vi "总氮流程质控自动启动.vi"(10 "总氮量程切换":enum32{"H", "L", "AUTO"}(ring)=enum."AUTO", 11 "参数":T1={"是否启用仪器"=FALSE, "CODMn"={"启动测量模式"={"测量模式"=enum."水样测量"}, "确定按钮"=TRUE}, "启动模块"={"氨氮"=FALSE, "总磷"=FALSE, "总氮"=FALSE, "COD"=FALSE}, "常规启动"=FALSE, "直接启动"=FALSE}) -> ()   [LabVIEW 2016]
panel:
  out "枚举 2":enum16{"初始化", "采配水启动", "等待", "配水", "排水", "结束"}(ring)
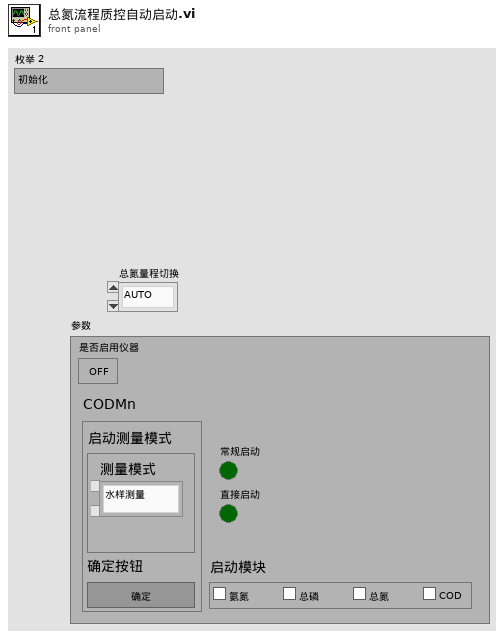
[diagram p1: front panel]
types:
  T1 = cluster{"是否启用仪器":bool, "CODMn":cluster{"启动测量模式":cluster{"测量模式":enum16{"水样测量", "标样核查", "加标回收", "平行样", "校零", "校标"}}, "确定按钮":bool}, "启动模块":cluster{"氨氮":bool, "总磷":bool, "总氮":bool, "COD":bool}, "常规启动":bool, "直接启动":bool}
  T2 = cluster{"R0":i16, "R1":i16, "R2":i16, "R3":i16, "R4":i16, "R5":i16, "R6":i16, "R7":i16, "R8":i16, "R9":i16, "R10":i16, "R11":i16, "R12":i16, "R13":i16, "R14":i16, "R15":i16, "R16":i16, "R17":i16, "R18":i16, "R19":i16, "R20":i16, "R21":i16, "R22":i16, "R23":i16, "R24":i16, "R25":i16, "R26":i16, "R27":i16, "R28":i16, "R29":i16, "R30":i16, "R31":i16, "R32":i16, "R33":i16, "R34":i16, "R35":i16, "R36":i16, "R37":i16, "R38":i16, "R39":i16, "R40":i16, "R41":i16, "R42":i16, "R43":i16, "R44":i16, "R45":i16, "R46":i16, "R47":i16, "R48":i16, "R49":i16, "R50":i16, "R51":i16, "R52":i16, "R53":i16, "R54":i16, "R55":i16, "R56":i16}
  T3 = enum32{"Bad", "Idle", "Run top level", "Running"}
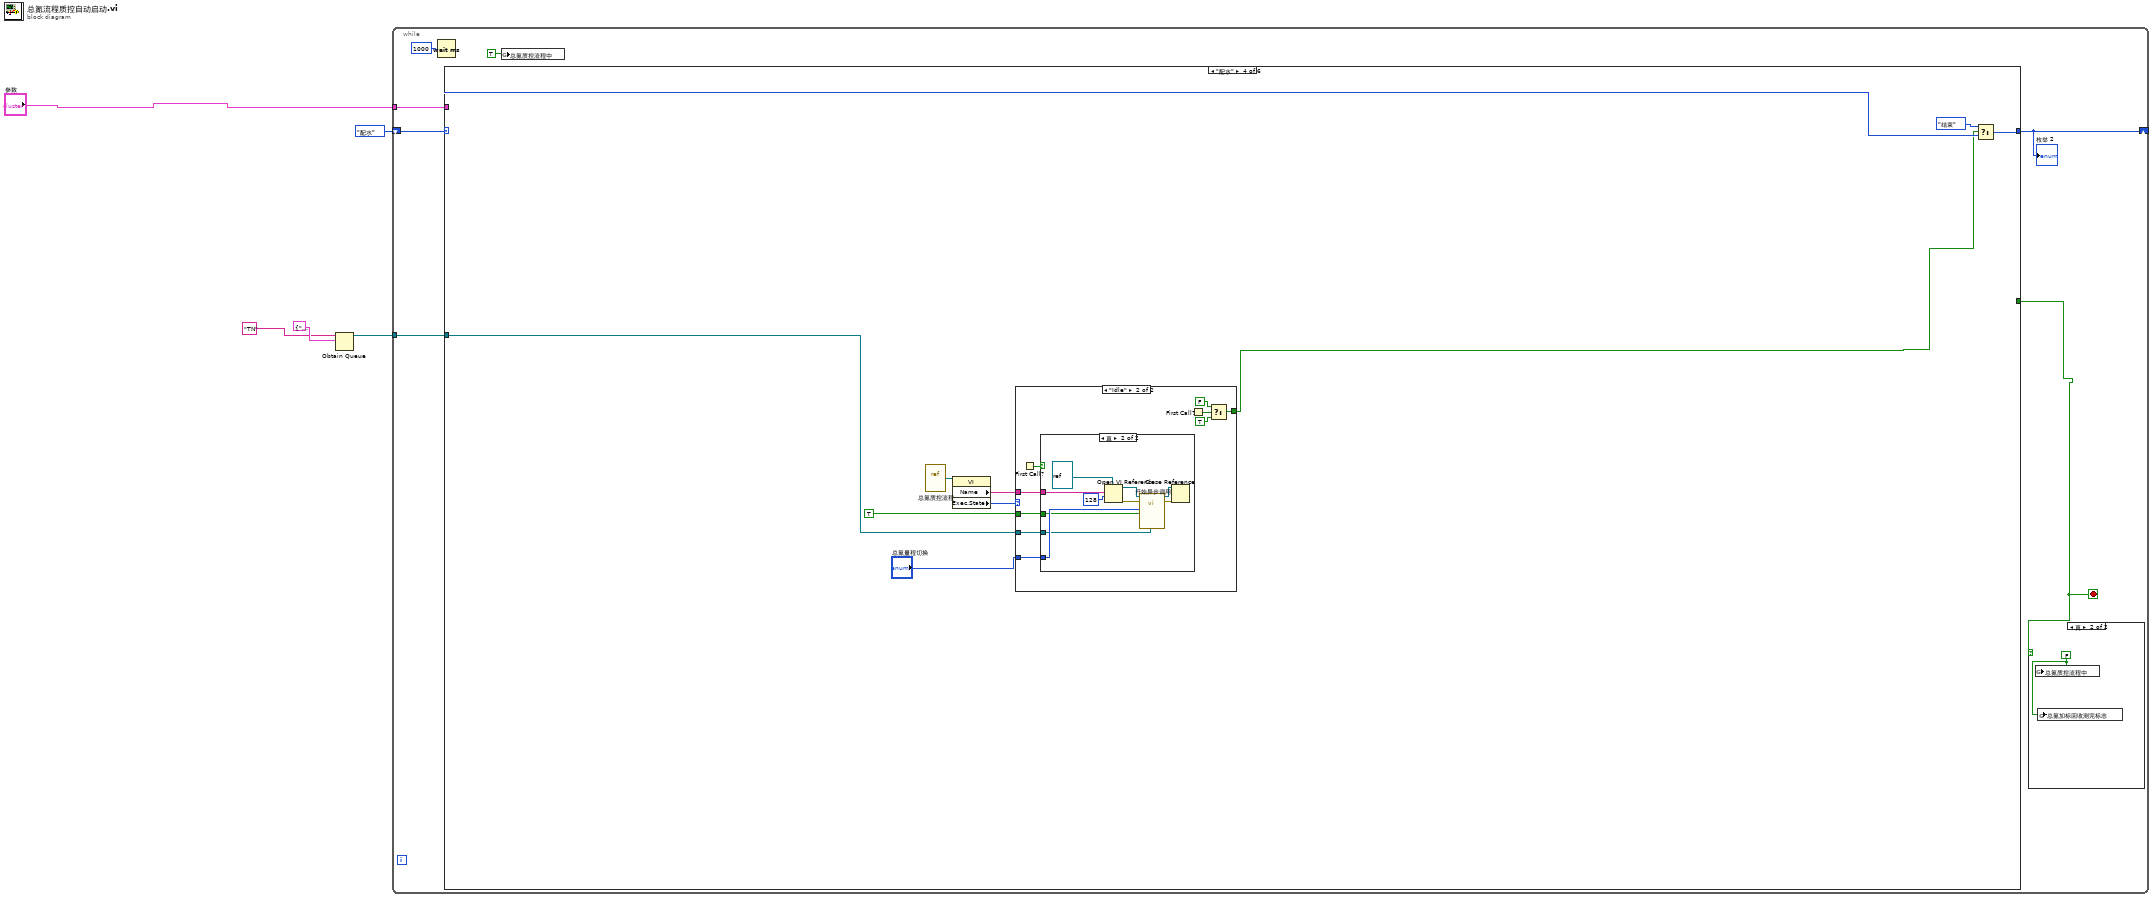
[diagram p0: block diagram]
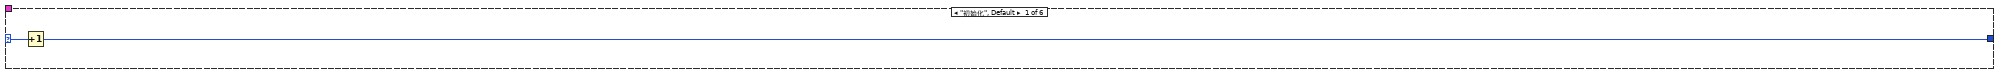
[diagram p3: hidden frame]
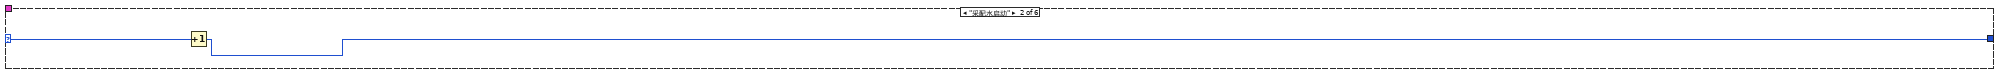
[diagram p4: hidden frame]
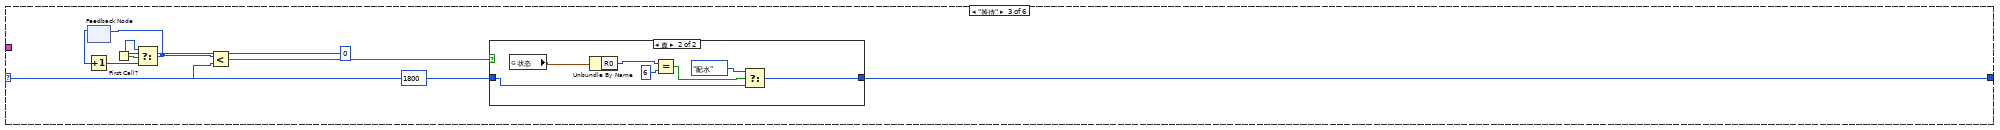
[diagram p5: hidden frame]
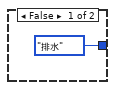
[diagram p6: hidden frame]
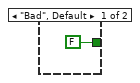
[diagram p7: hidden frame]
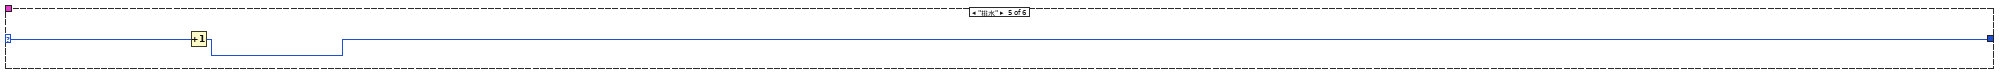
[diagram p9: hidden frame]
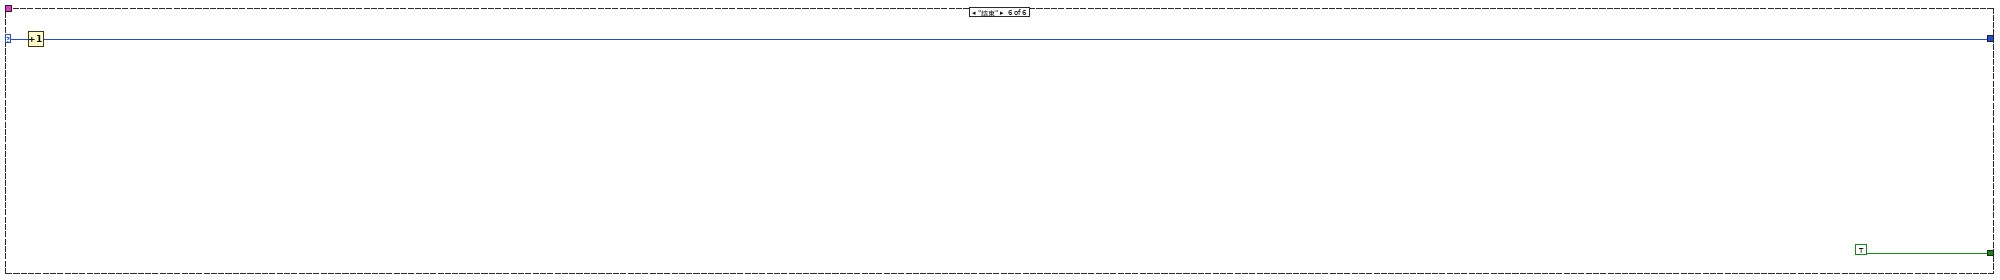
[diagram p10: hidden frame]
diagram:
  n1 = Obtain Queue(name (unnamed)="TN" ("名称（未命名）"), element data type=cluster{"命令":string, "data":variant} {"命令"="", "data"=variant}) -> (queue out=w1:refnum<queue>)  [unwired: 3 in, 2 out]
  n2 = while {
    shift-right: [w11] -> _
    shift-left: enum16{"初始化", "采配水启动", "等待", "配水", "排水", "结束"}."配水" ("枚举") -> [w12]
    tunnel: "参数" -> [w9]
    tunnel: w1 -> [w8]
    stop <- w6 stop-if-true
    n3 = Wait (ms)(milliseconds to wait=u32 1000 ("等待时间（毫秒）")) -> ()  [unwired: 1 out]
    n4 = case shown="\"配水\"" w12 {
      selector: w12 -> [w15 w17 w24 w43 w66 w69]
      tunnel: [w14 w16 w23 w42 w65 w68] -> w11
      tunnel: [_ _ _ _ _ TRUE] -> w6
      tunnel: w9 -> [_ _ _ _ _ _]
      tunnel: w8 -> [_ _ _ w37 _ _]
      frame "初始化", Default {
        n5 = Increment(x=w15) -> (x+1=w14:enum16{"初始化", "采配水启动", "等待", "配水", "排水", "结束"})
      }
      frame "采配水启动" {
        n6 = Increment(x=w17) -> (x+1=w16:enum16{"初始化", "采配水启动", "等待", "配水", "排水", "结束"})
      }
      frame "等待" {
        n7 = feedback #1() -> (w20:i32)  [unwired: 1 in]
        n8 = Increment(x=w20) -> (x+1=w19:i32)
        n9 = First Call?() -> (First Call?: T/F=w21:bool)
        n10 = Select(t=0, s=w21, f=w19) -> (s? t:f=w18:i32)
        n11 = feedback-in #1(w18) -> ()
        n12 = Less?(x=w18, y=1800) -> (x < y?=w25:bool)
        n13 = case shown="真" w25 {
          tunnel: w24 -> [_ w30]
          tunnel: [enum16{"初始化", "采配水启动", "等待", "配水", "排水", "结束"}."排水" ("枚举") w29] -> w23
          frame False {
          }
          frame True {
            n14 = global read "与采配水交互全局.vi" "状态"() -> (w28:T2)
            n15 = Unbundle By Name(w28) -> ("R0"=w34:i16)
            n16 = Equal?(x=w34, y=i16 6) -> (x = y?=w32:bool)
            n17 = Select(t=enum16{"初始化", "采配水启动", "等待", "配水", "排水", "结束"}."配水" ("枚举"), s=w32, f=w30) -> (s? t:f=w29:enum16{"初始化", "采配水启动", "等待", "配水", "排水", "结束"})
          }
        }
      }
      frame "配水" {
        n18 = vi-ref "总氮质控流程.vi"() -> (w40:refnum<vi>)
        n19 = property class="VI"(reference=w40) -> ("Name"=w41:string, "Exec.State"=w39:T3)  [unwired: 1 in, 2 out]
        n20 = case shown="\"Idle\"" w39 {
          tunnel: w41 -> [_ w54]
          tunnel: "总氮量程切换" -> [_ w53]
          tunnel: [FALSE w48] -> w35
          tunnel: TRUE -> [_ w47]
          tunnel: w37 -> [_ w46]
          frame "Bad", Default {
          }
          frame "Idle" {
            n21 = First Call?() -> (First Call?: T/F=w52:bool)
            n22 = case shown="真" w52 {
              tunnel: w54 -> [_ w64]
              tunnel: w53 -> [_ w58]
              tunnel: w47 -> [_ w57]
              tunnel: w46 -> [_ w56]
              frame False {
              }
              frame True {
                n23 = Open VI Reference(type specifier VI Refnum (for type only)=refnum<vi> refnum ("引用"), vi path=w64, options=128 ("选项")) -> (vi reference=w59:refnum<vi>, error out=w61:errorcluster)  [unwired: 3 in]
                n24 = call-by-ref "开始异步调用"(reference=w59, error in=w61, "队列输入TN"=w56, "总氮"=w57, "总氮量程切换"=w58) -> (reference out=w63:refnum<vi>, error out=w62:errorcluster)  [unwired: 6 in, 2 out]
                n25 = Close Reference(reference=w63, error in (no error)=w62) -> ()  [unwired: 1 out]
              }
            }
            n26 = First Call?() -> (First Call?: T/F=w51:bool)
            n27 = Select(t=FALSE, s=w51, f=TRUE) -> (s? t:f=w48:bool)
          }
        }
        n28 = Select(t=enum16{"初始化", "采配水启动", "等待", "配水", "排水", "结束"}."结束" ("枚举"), s=w35, f=w43) -> (s? t:f=w42:enum16{"初始化", "采配水启动", "等待", "配水", "排水", "结束"})
      }
      frame "排水" {
        n29 = Increment(x=w66) -> (x+1=w65:enum16{"初始化", "采配水启动", "等待", "配水", "排水", "结束"})
      }
      frame "结束" {
        n30 = Increment(x=w69) -> (x+1=w68:enum16{"初始化", "采配水启动", "等待", "配水", "排水", "结束"})
      }
    }
    "枚举 2" <- w11
    n31 = global write "质控测完标志全局 1.vi" "总氮质控流程中"(TRUE ("氨氮质控流程中")) -> ()
    n32 = case shown="真" w6 {
      frame False {
      }
      frame True {
        w13 = FALSE ("氨氮质控流程中")
        n33 = global write "质控测完标志全局 1.vi" "总氮质控流程中"(w13) -> ()
        n34 = global write "质控测完标志全局 1.vi" "总氮加标回收测完标志"(w13) -> ()
      }
    }
  }
